vi "readTimeMark.vi"(8 "Error In":errorcluster, 11 "FGV_data":T2) -> (0 "Error Out":errorcluster, 2 "data":T1[](array[typedef]), 3 "FGV_data out":T2)   [LabVIEW 2018]
uses:
  FGV_data.ctl
  Config/config_data.ctl
  AE/timeMark_data.ctl
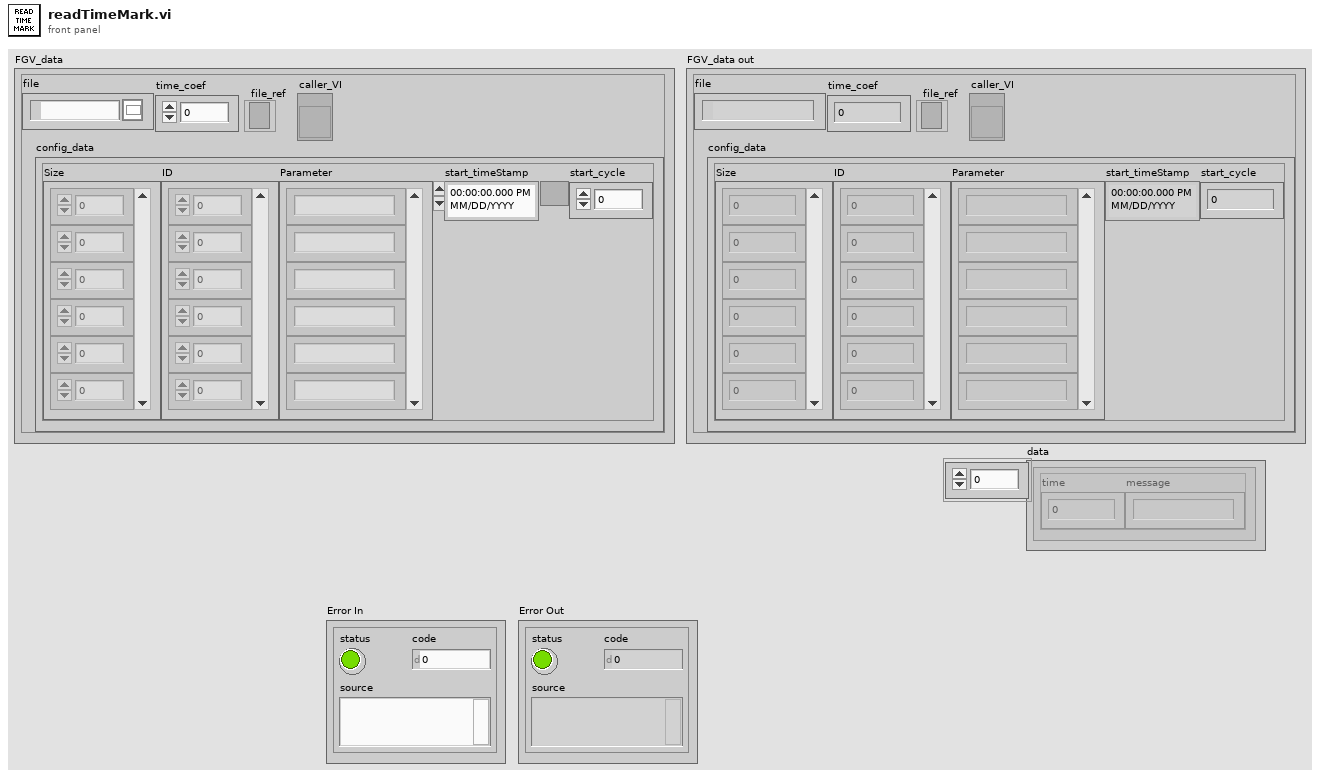
[diagram p1: front panel]
types:
  T1 = typedef "timeMark_data.ctl" = cluster{"time":dbl, "message":string}
  T2 = typedef "FGV_data.ctl" = cluster{"file":path, "time_coef":dbl, "config_data":T3, "file_ref":refnum<file>, "caller_VI":refnum<vi>}
  T3 = typedef "config_data.ctl" = cluster{"Size":i32[], "ID":u8[], "Parameter":string[], "start_timeStamp":timestamp, "start_cycle":u64}
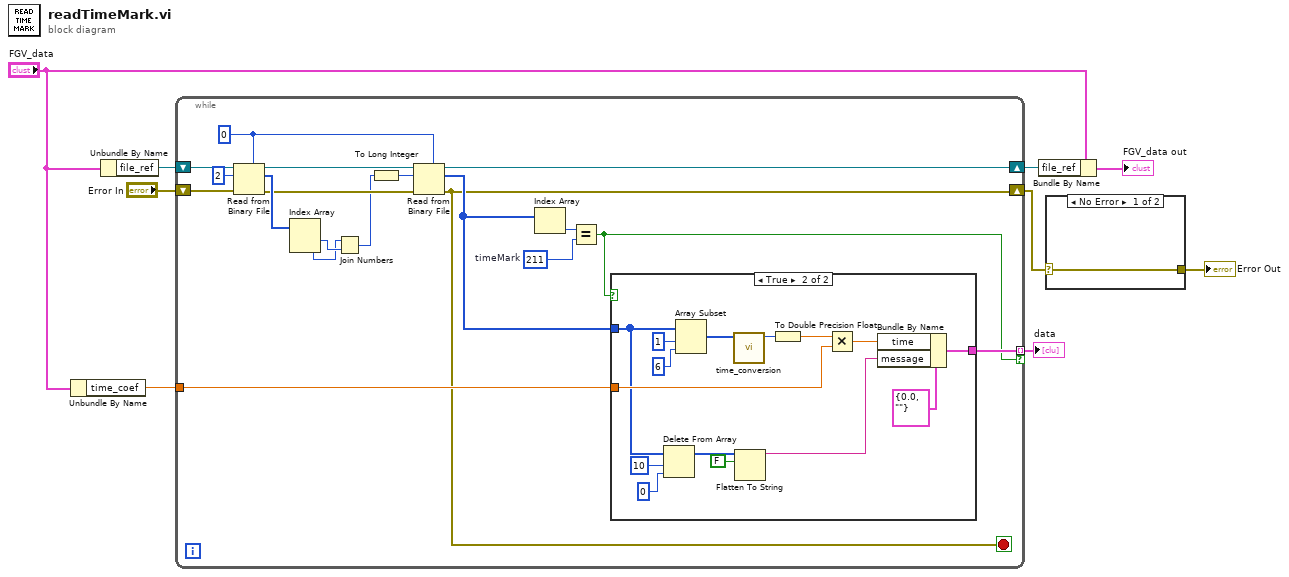
[diagram p0: block diagram]
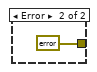
[diagram p3: hidden frame]
diagram:
  n1 = Unbundle By Name("FGV_data") -> ("time_coef"=w4:dbl)
  n2 = Unbundle By Name("FGV_data") -> ("file_ref"=w9:refnum<file>)
  n3 = while {
    shift-right: [w12] -> w3
    shift-left: "Error In" -> [w20]
    shift-right: [w15] -> w7
    shift-left: w9 -> [w28]
    tunnel: w4 -> [w14]
    tunnel: [w11] -> w1 mode=indexing if=w10
    stop <- w12 stop-if-true
    w17 = u8 211  # timeMark
    w23 = u8 0
    n4 = Read from Binary File(5:w23, 8:w20, 10:2 ("count (1)"), 11:w28) -> (0:w24:errorcluster, 2:w26:u8[], 3:w25:refnum<file>)  [unwired: 2 in, 1 out]
    n5 = Index Array(array=w26) -> (element #1=w22:u8, element #2=w21:u8)  [unwired: 2 in]
    n6 = Join Numbers(hi=w21, lo=w22) -> ((hi.lo)=w19:u16)
    n7 = To Long Integer(number=w19) -> (32bit integer=w18:i32)
    n8 = Read from Binary File(5:w23, 8:w24, 10:w18, 11:w25) -> (0:w12:errorcluster, 2:w13:u8[], 3:w15:refnum<file>)  [unwired: 2 in, 1 out]
    n9 = Index Array(array=w13) -> (element=w16:u8)  [unwired: 1 in]
    n10 = Equal?(x=w16, y=w17) -> (x = y?=w10:bool)
    n11 = case shown="True" w10 {
      tunnel: w13 -> [_ w35]
      tunnel: w14 -> [_ w36]
      tunnel: [_ w29] -> w11
      frame False {
      }
      frame True {
        n12 = Delete From Array(array=w35, length=10 ("inicial"), index=0) -> (array with subset deleted=w34:u8[])  [unwired: 1 out]
        n13 = Array Subset(array=w35, index=1, length=6) -> (w38:u8[])
        n14 = call "time_conversion.vi"("array_time"=w38) -> ("time_U64"=w37:u64)  [unwired: 10 in]
        n15 = Flatten To String(anything=w34, prepend array or string size? (T)=FALSE) -> (data string=w30:string)  [unwired: 2 in, 2 out]
        n16 = To Double Precision Float(number=w37) -> (double precision float=w39:dbl)
        n17 = Multiply(x=w39, y=w36) -> (x*y=w31:dbl)
        n18 = Bundle By Name(cluster=T1 {"time"=0.0, "message"=""} ("timeMark_data"), "time"=w31, "message"=w30) -> (w29:T1)
      }
    }
  }
  "data" <- w1
  n19 = Bundle By Name(cluster="FGV_data", "file_ref"=w7) -> (→"FGV_data out":T2)
  n20 = case shown="No Error" w3 {
    selector: w3 -> [w44 _]
    tunnel: [w44 errorcluster {"status"=FALSE, "code"=0, "source"=""} ("error IO")] -> w2
    frame No Error {
    }
    frame Error {
    }
  }
  "Error Out" <- w2
